vi "Launch as Nested.vi"(6 "Wait to Start (F)":bool, 8 "error in (no error)":errorcluster, 10 "Test 1 (New)":refnum<class "Test 1.lvclass">, 11 "Caller In":refnum<class "Actor.lvclass">) -> (0 "error out":errorcluster, 2 "Test 1 API":refnum<class "Test 1 API.lvclass">, 3 "Caller":refnum<class "Actor.lvclass">)   [LabVIEW 2020, in "Scratchpad.lvlib" / "Test 1.lvlib" / "Test 1.lvclass"]
uses:
  Test 1.lvclass
  Artifex/Actor/Actor.lvclass
  Test 1 API/Test 1 API.lvclass
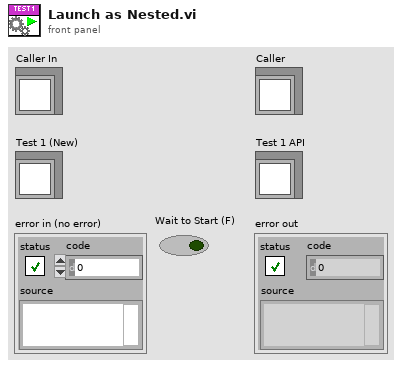
[diagram p1: front panel]
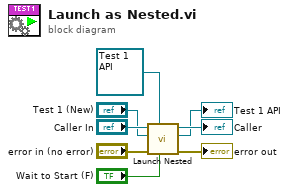
[diagram p0: block diagram]
diagram:
  n1 = call "Launch Nested.vi"("Wait to Start (F)"="Wait to Start (F)", "API Type (Base)"=refnum<class "Test 1 API.lvclass"> refnum ("Scratchpad.lvlib:Test 1.lvlib:Test 1 API.lvclass"), "error in (no error)"="error in (no error)", "Nested Actor"="Test 1 (New)", "Actor in"="Caller In") -> ("error out"=→"error out":errorcluster, "Nested API"=→"Test 1 API":refnum<class "Test 1 API.lvclass">, "Actor out"=→"Caller":refnum<class "Actor.lvclass">)  [unwired: 4 in]
